vi "UIRef.vi"(8 "error in":errorcluster, 11 "node in":refnum<class "VI modification.lvclass">) -> (0 "error out":errorcluster, 2 "VI refnum":refnum<vi>, 3 "node out":refnum<class "VI modification.lvclass">)   [LabVIEW 2013, in "VI modification.lvclass"]
doc: "Stores the static reference to the UI of the node."
uses:
  VI modification.lvclass
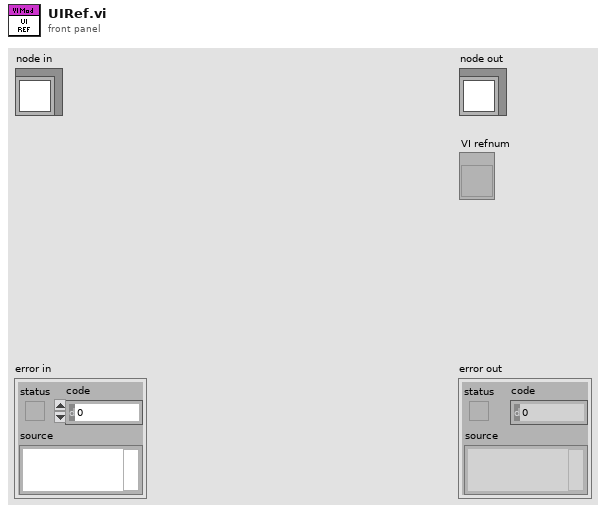
[diagram p1: front panel]
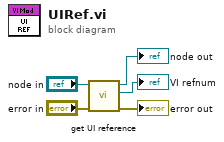
[diagram p0: block diagram]
diagram:
  n1 = call-dynamic "get UI reference.vi"("error in"="error in", "VI modification in"="node in") -> ("error out"=→"error out":errorcluster, "VI Refnum"=→"VI refnum":refnum<vi>, "VI modification out"=→"node out":refnum<class "VI modification.lvclass">)  [unwired: 7 in]
